vi "HEWH RLT Update AGILENT Channels.vi"(8 "Error In":errorcluster, 9 "Channel":string, 10 "Label":string, 11 "Station A in":T1) -> (0 "Error Out":errorcluster, 3 "Station A out":T1)   [LabVIEW 2016]
uses:
  Type Definitions/HEWH RLT Stations.ctl
  Type Definitions/HEWH Label Channel.ctl
  Custom Instrument Control/MW100/Type Definitions/HEWH MW100 Channel Numbers.ctl
  Type Definitions/PRAT Channel Settings.ctl
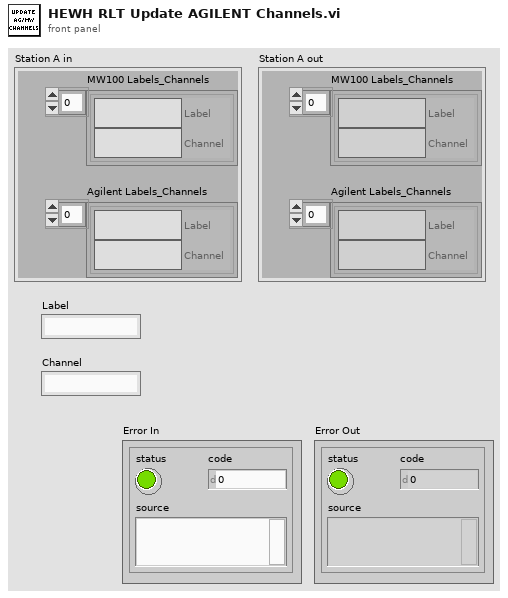
[diagram p1: front panel]
types:
  T1 = typedef "HEWH RLT Stations.ctl" = cluster{"MW100 Labels_Channels":T2[], "Agilent Labels_Channels":T2[]}
  T2 = typedef "HEWH Label Channel.ctl" = cluster{"Label":string, "Channel":string}
  T3 = typedef "PRAT Channel Settings.ctl" = string
  T4 = typedef "HEWH MW100 Channel Numbers.ctl" = string
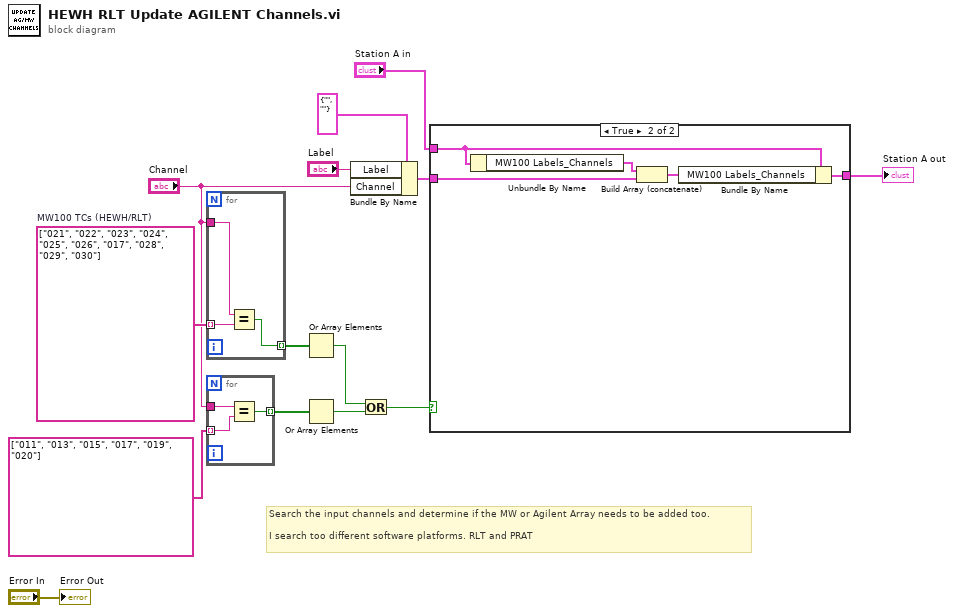
[diagram p0: block diagram]
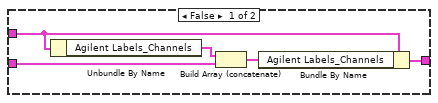
[diagram p2: hidden frame]
diagram:
  w8 = T4[] ["021", "022", "023", "024", "025", "026", "017", "028", "029", "030"]  # MW100 TCs (HEWH/RLT)
  # "Search the input channels and determine if the MW or Agilent Array needs to be added too.\n\nI search too different software platforms. RLT and PRAT"
  n1 = for {
    tunnel: w8 -> [w16] mode=indexing
    tunnel: "Channel" -> [w17]
    tunnel: [w15] -> w7 mode=indexing
    n2 = Equal?(x=w17, y=w16) -> (x = y?=w15:bool)
  }
  n3 = for {
    tunnel: T3[] ["011", "013", "015", "017", "019", "020"] -> [w19] mode=indexing
    tunnel: "Channel" -> [w20]
    tunnel: [w18] -> w5 mode=indexing
    n4 = Equal?(x=w20, y=w19) -> (x = y?=w18:bool)
  }
  n5 = Or Array Elements(Boolean array=w7) -> (logical OR=w4:bool)
  n6 = Or Array Elements(Boolean array=w5) -> (logical OR=w3:bool)
  n7 = Bundle By Name(cluster=T2 {"Label"="", "Channel"=""} ("input cluster"), "Label"="Label", "Channel"="Channel") -> (w12:T2)
  n8 = Or(x=w4, y=w3) -> (x .or. y?=w2:bool)
  n9 = case shown="True" w2 {
    tunnel: [w25 w27] -> w14
    tunnel: "Station A in" -> [w24 w28]
    tunnel: w12 -> [w22 w26]
    frame False {
      n10 = Unbundle By Name(w24) -> ("Agilent Labels_Channels"=w21:T2[])
      n11 = Build Array (concatenate)(w21, w22) -> (w23:T2[])
      n12 = Bundle By Name(cluster=w24, "Agilent Labels_Channels"=w23) -> (w25:T1)
    }
    frame True {
      n13 = Unbundle By Name(w28) -> ("MW100 Labels_Channels"=w29:T2[])
      n14 = Build Array (concatenate)(w29, w26) -> (w30:T2[])
      n15 = Bundle By Name(cluster=w28, "MW100 Labels_Channels"=w30) -> (w27:T1)
    }
  }
  "Station A out" <- w14
  "Error Out" <- "Error In"
